vi "Test USB NavX.vi"() -> ()   [LabVIEW 2014]
uses:
  navX-MXP Library/COMMON/TypeDefs/navX YPRH Data.ctl
  navX-MXP Library/SERIAL/TypeDefs/navX Serial Mode.ctl
  navX-MXP Library/SERIAL/IO/NI WPI/WPI_SerialPort_USB.ctl
  navX-MXP Library/navX-MXP IMU.lvlib
panel:
  out "Numeric":i32
  out "YPRH":T1
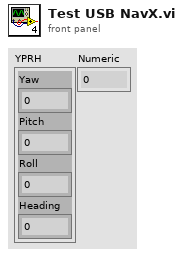
[diagram p1: front panel]
types:
  T1 = typedef "navX-MXP IMU.lvlib/navX YPRH Data.ctl" = cluster{"Yaw":dbl, "Pitch":dbl, "Roll":dbl, "Heading":dbl}
  T2 = typedef "navX-MXP IMU.lvlib/WPI_SerialPort_USB.ctl" = enum16{"Onboard RS-232", "MXP TTL", "USB"}
  T3 = typedef "navX-MXP IMU.lvlib/navX Serial Mode.ctl" = enum16{"YPR", "Gyro", "Quaternion"}
  T4 = typedef "navX-MXP IMU.lvlib/navX Serial DevRef.ctl" = cluster{"SerialPortRef":T5, "Board Information":T6, "Status":T7, "Offsets":cluster{"Yaw":dbl, "Quat W":dbl, "Quat X":dbl, "Quat Y":dbl, "Quat Z":dbl}, "Update Rate (4Hz-60Hz)":u8, "Nav6Mode (YPR)":T3, "refnum name":string, "error":errorcluster}
  T5 = typedef "WPI_SerialPortRef.ctl" = cluster{"DevStatus":errorcluster, "Serial Port Name":refnum<visa-resource-name>}
  T6 = typedef "navX-MXP IMU.lvlib/navX Board Information.ctl" = cluster{"WhoAmI (50 | 0x32)":u8, "Board Revision":u8, "Firmware Major Version":u8, "Firmware Minor Version":u8}
  T7 = typedef "navX-MXP IMU.lvlib/navX Status Data.ctl" = cluster{"Update Rate Hz":u8, "Accelerometer Full-Scale Range":u8, "Gyro Full-Scale Range":u16, "NAVX_OP_STATUS":T8, "NAVX_CAL_STATUS":T9, "NAVX_SELFTEST_STATUS":u8, "NAVX_SENSOR_STATUS":T10}
  T8 = typedef "navX-MXP IMU.lvlib/navX NAVX_OP_STATUS.ctl" = u8
  T9 = typedef "navX-MXP IMU.lvlib/navX NAVX_CAL_STATUS.ctl" = u8
  T10 = typedef "navX-MXP IMU.lvlib/navX NAVX_SENSOR_STATUS.ctl" = cluster{"MOVING":bool, "YAW_STABLE":bool, "MAG_DISTURBANCE":bool, "ALTITUDE_VALID":bool, "SEALEVEL_PRESS_SET":bool, "FUSED_HEADING_VALID":bool}
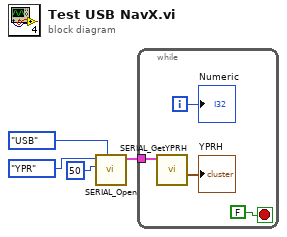
[diagram p0: block diagram]
diagram:
  n1 = call "SERIAL_Open.vi"("Serial Port (MXP)"=WPI_SerialPort_USB."USB", "Update Rate (4Hz-60Hz)"=u8 50, "Nav6Mode (YPR)"=navX_Serial_Mode."YPR") -> ("navX Ref"=w1:T4)  [unwired: 6 in, 2 out]
  n2 = while {
    tunnel: w1 -> [w8]
    i -> [w5]
    stop <- FALSE stop-if-true
    n3 = call "SERIAL_GetYPRH.vi"("navX Ref Object"=w8) -> ("YPRH"=→"YPRH":T1)  [unwired: 9 in, 1 out]
    "Numeric" <- w5
  }
